vi "Get Default Step Settings.vi"(11 "UI Data In":refnum<class "Settings UI.lvclass">) -> (2 "Default Step Settings":T1, 3 "UI Data out":refnum<class "Settings UI.lvclass">)   [LabVIEW 2020, in "Output Sequencer.lvlib" / "Settings UI.lvclass"]
uses:
  Settings UI.lvclass
  Types/Step Settings.ctl
  Output Sequencer/Globals/Global Strings.vi
  Output Sequencer/Output Sequencer.lvclass
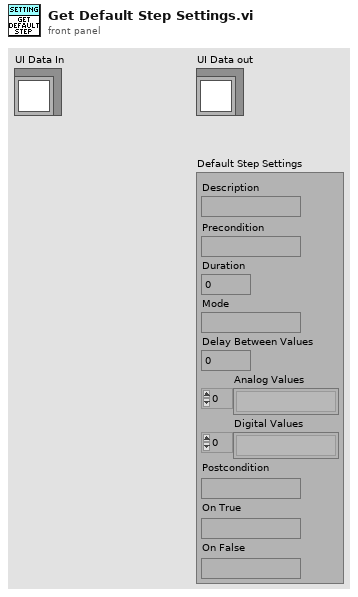
[diagram p1: front panel]
types:
  T1 = typedef "Output Sequencer.lvlib/Settings UI.lvclass/Step Settings.ctl" = cluster{"Description":string, "Precondition":string, "Duration":dbl, "Mode":string, "Delay Between Values":dbl, "Analog Values":string[], "Digital Values":string[], "Postcondition":string, "On True":string, "On False":string}
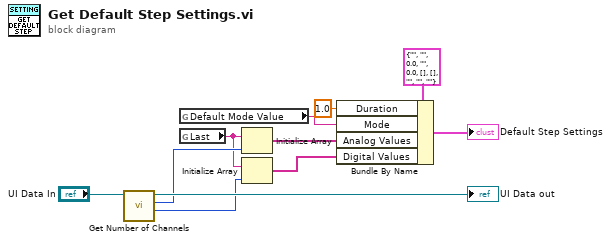
[diagram p0: block diagram]
diagram:
  n1 = call "Get Number of Channels.vi"("UI Data In"="UI Data In") -> ("Num of Digital Channels"=w6:i32, "Num of Analog Channels"=w4:i32, "UI Data out"=→"UI Data out":refnum<class "Settings UI.lvclass">)  [unwired: 7 in, 1 out]
  n2 = global read "Global Strings.vi" "Default Mode Value"() -> (w10:string)
  n3 = global read "Global Strings.vi" "Last"() -> (w2:string)
  n4 = Initialize Array(w2, w4) -> (w3:string[])
  n5 = Initialize Array(w2, w6) -> (w5:string[])
  n6 = Bundle By Name(cluster=T1 {"Description"="", "Precondition"="", "Duration"=0.0, "Mode"="", "Delay Between Values"=0.0, "Analog Values"=[], "Digital Values"=[], "Postcondition"="", "On True"="", "On False"=""} ("Step Settings"), "Duration"=1.0, "Mode"=w10, "Analog Values"=w3, "Digital Values"=w5) -> (→"Default Step Settings":T1)
